vi "DAQ.Start.AO.vi"(8 "error in (no error)":errorcluster, 10 "AO []":waveform(dbl)[](array[waveform]), 11 "Instrument.DAQ in":refnum<class "Instrument.DAQ.lvclass">) -> (0 "error out":errorcluster, 3 "Instrument.DAQ out":refnum<class "Instrument.DAQ.lvclass">)   [LabVIEW 2019, in "Instrument.Lockin.lvlib" / "Instrument.DAQ.lvclass"]
uses:
  Instrument.DAQ.lvclass
  Instrument.DAQ.lvclass/Instrument.DAQ.ctl
  <resource>/objmgr/daqmx.rc
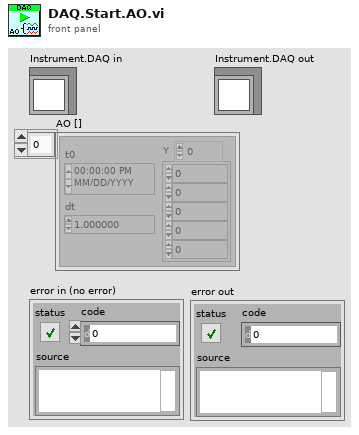
[diagram p1: front panel]
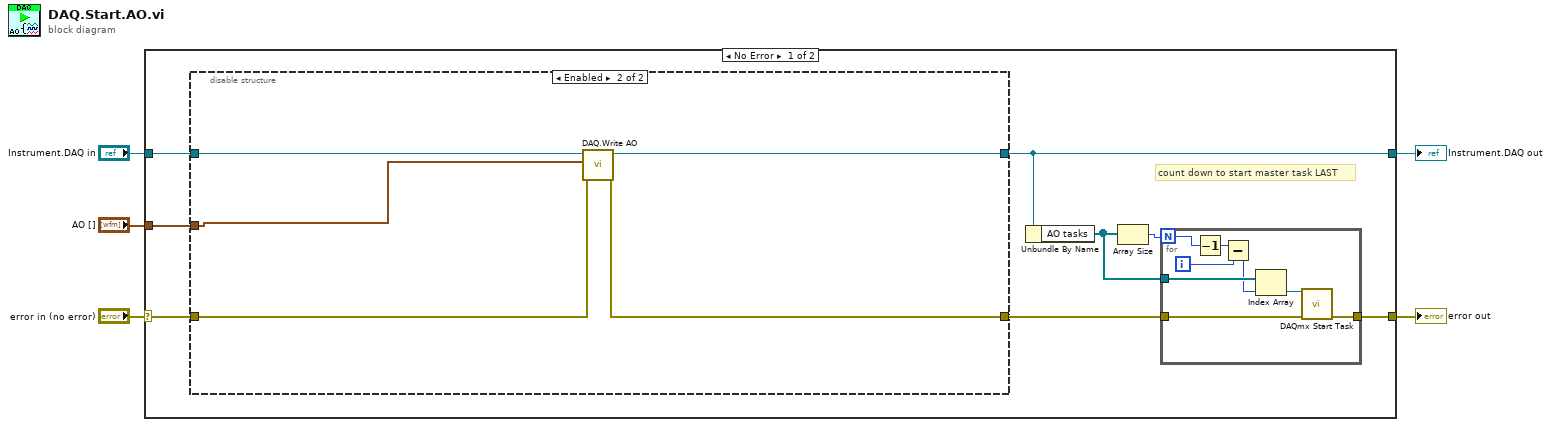
[diagram p0: block diagram]
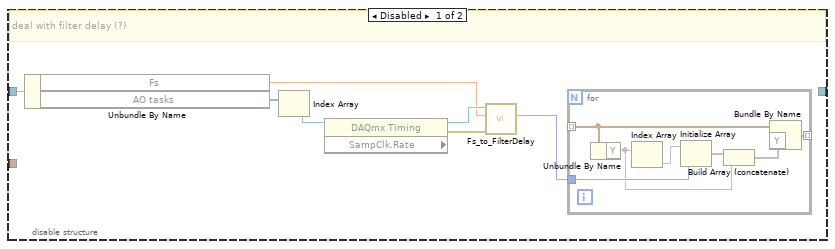
[diagram p2: hidden frame]
diagram:
  n1 = case shown="No Error" "error in (no error)" {
    selector: "error in (no error)" -> [w10 w43]
    tunnel: [w13 w43] -> w5
    tunnel: "Instrument.DAQ in" -> [w9 w42]
    tunnel: [w7 w42] -> w2
    tunnel: "AO []" -> [w6 _]
    frame No Error {
      # "count down to start master task LAST"
      n2 = disable-structure shown="Enabled" {
        disable-tunnel: w9 -> [w14 w31]
        disable-tunnel: w10 -> [_ w30]
        disable-tunnel: [_ w32] -> w8
        disable-tunnel: [_ w33] -> w7
        disable-tunnel: w6 -> [_ w29]
        frame Disabled {
          # "deal with filter delay (?)"
          n3 = Unbundle By Name(w14) -> ("Fs"=w17:dbl, "AO tasks"=w19:refnum<k21>[])
          n4 = Index Array(array=w19) -> (element=w16:refnum<k21>)  [unwired: 1 in]
          n5 = property class="DAQmx Timing" props=["SampClk.Rate"](reference=w16) -> (reference out=w21:refnum<k21>, error in=w15:errorcluster, error out=w20:errorcluster)  [unwired: 1 out]
          n6 = call "Fs_to_FilterDelay.vi"("error in (no error)"=w20, "Fs"=w17, "Refnum in"=w21) -> ("Total Filter Delay (samples)"=w18:i32)  [unwired: 6 in, 2 out]
          n7 = for {
            tunnel: _ -> [w23] mode=indexing
            tunnel: w18 -> [w27]
            tunnel: [w22] -> _ mode=indexing
            n8 = Unbundle By Name(w23) -> ("Y"=w25)
            n9 = Index Array(array=w25) -> (element=w28)  [unwired: 1 in]
            n10 = Initialize Array(w28, w27) -> (w26:void[])
            n11 = Build Array (concatenate)(w26, w25) -> (w24:void[])
            n12 = Bundle By Name(cluster=w23, "Y"=w24) -> (w22:waveform(dbl))
          }
        }
        frame Enabled {
          n13 = call "DAQ.Write AO.vi"("error in (no error)"=w30, "AO []"=w29, "Instrument.DAQ in"=w31) -> ("error out"=w32:errorcluster, "Instrument.DAQ out"=w33:refnum<class "Instrument.DAQ.lvclass">)  [unwired: 5 in, 2 out]
        }
      }
      n14 = Unbundle By Name(w7) -> ("AO tasks"=w12:refnum<k21>[])
      n15 = Array Size(array=w12) -> (size(s)=w11:i32)
      n16 = for {
        N: w11 -> [w38]
        tunnel: w12 -> [w40]
        tunnel: [w41] -> w13
        tunnel: w8 -> [w34]
        i -> [w35]
        n17 = Decrement(x=w38) -> (x-1=w37:i32)
        n18 = Subtract(x=w37, y=w35) -> (x-y=w36:i32)
        n19 = Index Array(array=w40, index=w36) -> (element=w39:refnum<k21>)
        n20 = call <vilib>:"DAQmx Start Task.vi"("task/channels in"=w39, "error in"=w34) -> ("error out"=w41:errorcluster)  [unwired: 12 in, 1 out]
      }
    }
    frame Error {
    }
  }
  "Instrument.DAQ out" <- w2
  "error out" <- w5
